vi "Helmholtz2D_FEM_Assemble_RHS.vi"(4 "a":dbl, 5 "F(x, y)":dbl[](array[numeric]), 6 "k":dbl, 7 "# of unknown":i32, 8 "Mass Mtrx":dbl[][](array[numeric]), 9 "Stiffness Mtrx":dbl[][](array[numeric]), 10 "Triangle":i32[](array[numeric]), 11 "RHS In":dbl[](array[numeric])) -> (3 "RHS Out":dbl[](array[numeric]))   [LabVIEW 2020, in "NI_PDE.lvlib"]
uses:
  <vilib>/gmath/NI_PDE.lvlib
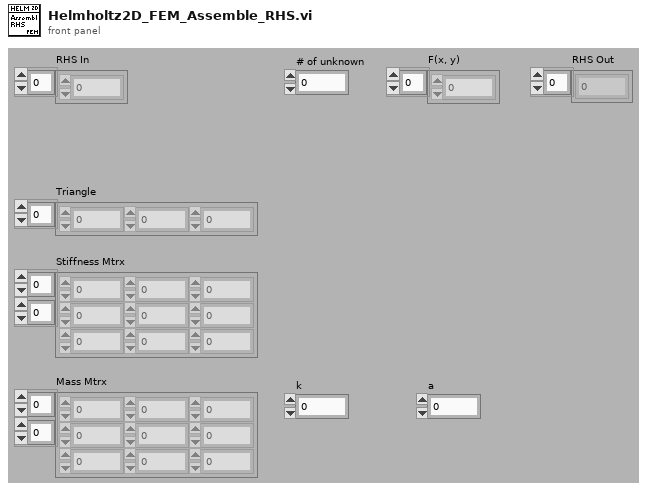
[diagram p1: front panel]
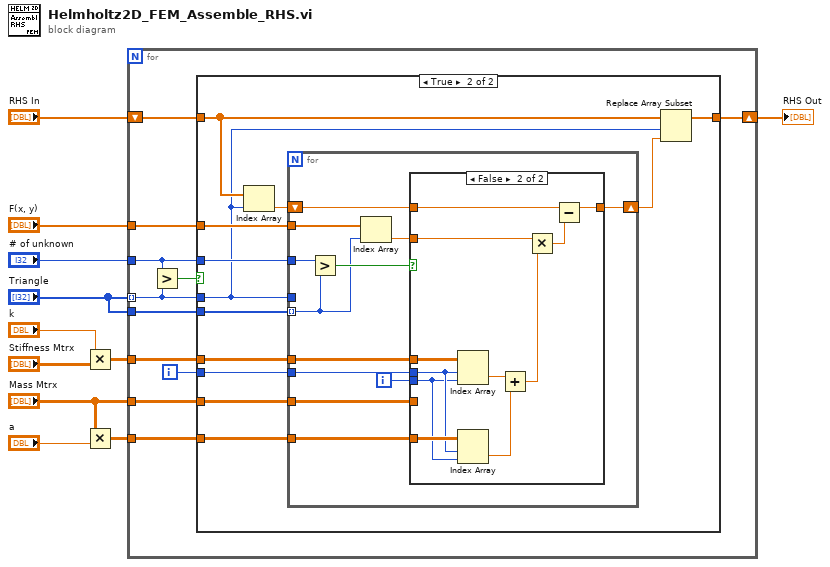
[diagram p0: block diagram]
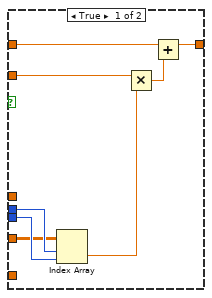
[diagram p3: hidden frame]
diagram:
  n1 = Multiply(x="k", y="Stiffness Mtrx") -> (x*y=w7:dbl[][])
  n2 = Multiply(x="Mass Mtrx", y="a") -> (x*y=w6:dbl[][])
  n3 = for {
    tunnel: "Triangle" -> [w14] mode=indexing
    tunnel: "Triangle" -> [w22]
    tunnel: w7 -> [w21]
    tunnel: w6 -> [w20]
    tunnel: "Mass Mtrx" -> [w19]
    shift-right: [w17] -> w3
    shift-left: "RHS In" -> [w18]
    tunnel: "# of unknown" -> [w13]
    tunnel: "F(x, y)" -> [w16]
    i -> [w15]
    n4 = Greater?(x=w13, y=w14) -> (0:w12:bool)
    n5 = case shown="True" w12 {
      tunnel: w22 -> [_ w35]
      tunnel: w21 -> [_ w34]
      tunnel: w20 -> [_ w33]
      tunnel: w19 -> [_ w32]
      tunnel: w18 -> [w23 w27]
      tunnel: [w23 w26] -> w17
      tunnel: w16 -> [_ w31]
      tunnel: w15 -> [_ w30]
      tunnel: w14 -> [_ w24]
      tunnel: w13 -> [_ w29]
      frame False {
      }
      frame True {
        n6 = Index Array(array=w27, index=w24) -> (element=w28:dbl)
        n7 = for {
          tunnel: w35 -> [w37] mode=indexing
          tunnel: w24 -> [_]
          tunnel: w34 -> [w45]
          tunnel: w33 -> [w43]
          tunnel: w32 -> [w44]
          tunnel: w29 -> [w47]
          tunnel: w31 -> [w38]
          tunnel: w30 -> [w42]
          shift-right: [w39] -> w25
          shift-left: w28 -> [w40]
          i -> [w41]
          n8 = Greater?(x=w47, y=w37) -> (0:w46:bool)
          n9 = Index Array(array=w38, index=w37) -> (element=w36:dbl)
          n10 = case shown="False" w46 {
            tunnel: w45 -> [_ w64]
            tunnel: w44 -> [w53 _]
            tunnel: w43 -> [_ w62]
            tunnel: w42 -> [w55 w61]
            tunnel: w41 -> [w54 w60]
            tunnel: w40 -> [w51 w66]
            tunnel: [w49 w65] -> w39
            tunnel: w36 -> [w48 w57]
            frame True {
              n11 = Index Array(array=w53, index (row)=w55, index (col)=w54) -> (element=w52:dbl)
              n12 = Multiply(x=w48, y=w52) -> (x*y=w50:dbl)
              n13 = Add(x=w51, y=w50) -> (x+y=w49:dbl)
            }
            frame False {
              n14 = Index Array(array=w64, index (row)=w61, index (col)=w60) -> (element=w63:dbl)
              n15 = Index Array(array=w62, index (row)=w61, index (col)=w60) -> (element=w59:dbl)
              n16 = Add(x=w63, y=w59) -> (x+y=w58:dbl)
              n17 = Multiply(x=w57, y=w58) -> (x*y=w56:dbl)
              n18 = Subtract(x=w66, y=w56) -> (x-y=w65:dbl)
            }
          }
        }
        n19 = Replace Array Subset(array=w27, new element=w25, index=w24) -> (w26:dbl[])
      }
    }
  }
  "RHS Out" <- w3
